vi "AO_arbitrary.vi"() -> ()   [LabVIEW 2021]
uses:
  <vilib>/userdefined/High Color/nirio_resource_hc.ctl
  <vilib>/FPGAPlugInAG/PCIe-7857/niLvFpga_Open_PCIe-7857.vi
  <vilib>/Utility/error.llb/Error Cluster From Error Code.vi
  <vilib>/rvi/errors/niLvFpgaAdjustHostInterfaceError.vi
  <vilib>/rvi/interface/common/niFpgaWaitOnOcc.vi
  <vilib>/FPGAPlugInAG/PCIe-7857/niLvFpga_Run_PCIe-7857.vi
  <vilib>/FPGAPlugInAG/PCIe-7857/niLvFpga_Close_PCIe-7857.vi
  <vilib>/rvi/interface/nirviOpenFPGA/nirviOpenFPGA.xnode
  FPGA Bitfiles/lvfpga2_FPGATarget_FPGA_J9MBVCOB9rw.lvbitx
  FPGA.vi
  <vilib>/rvi/interface/nirviReadWriteControl/nirviReadWriteControl.xnode
  <vilib>/rvi/interface/nirviMethod/nirviMethod.xnode
  <vilib>/rvi/interface/nirviCloseFPGA/nirviCloseFPGA.xnode
  <vilib>/rvi/errors/niLvFpgaMergeErrorWithErrorCode.vi
  <vilib>/measure/NI_MABase.lvlib
  <vilib>/FPGAPlugInAG/PCIe-7857/niLvFpga_WriteFifo_PCIe-7857.vi
  <vilib>/FPGAPlugInAG/PCIe-7857/niLvFpga_ConfigureFifo_PCIe-7857.vi
  NiFpgaLv.dll
panel:
  out "Actual Depth":u32
  out "Waveform Graph 2":dbl[](graph)
  out "Waveform Graph":waveform(dbl)(graph)
  in  "RIO Resource Name":T1="RIO0" caption="RIO Device"
  in  "Sample Clock Rate":dbl=20000.0 format="%0.2f"
  in  "stop":bool
  out "Actual Sample Clock Rate":dbl=20000.0 format="%.2f"
  in  "Size (Samples)":u32=5000
  in  "Waveform Type":T2(ring)
  in  "Frequency":sgl=997.0 format="%.2f"
  in  "Amplitude":sgl=1.0 format="%0.2p"
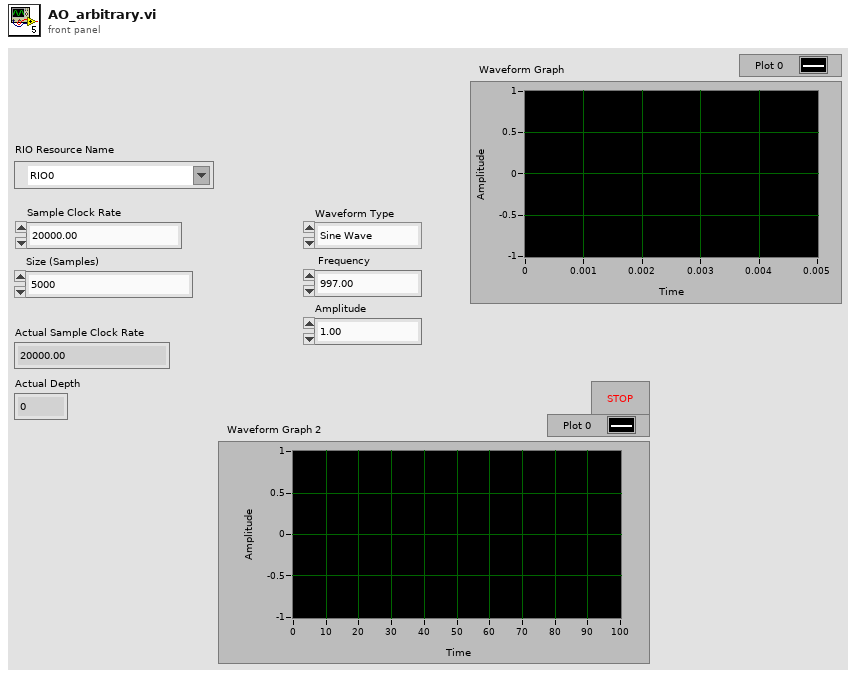
[diagram p1: front panel]
types:
  T1 = typedef "nirio_resource_hc.ctl" = tag
  T2 = enum16{"Sine Wave", "Triangle Wave", "Square Wave", "Sawtooth Wave"}
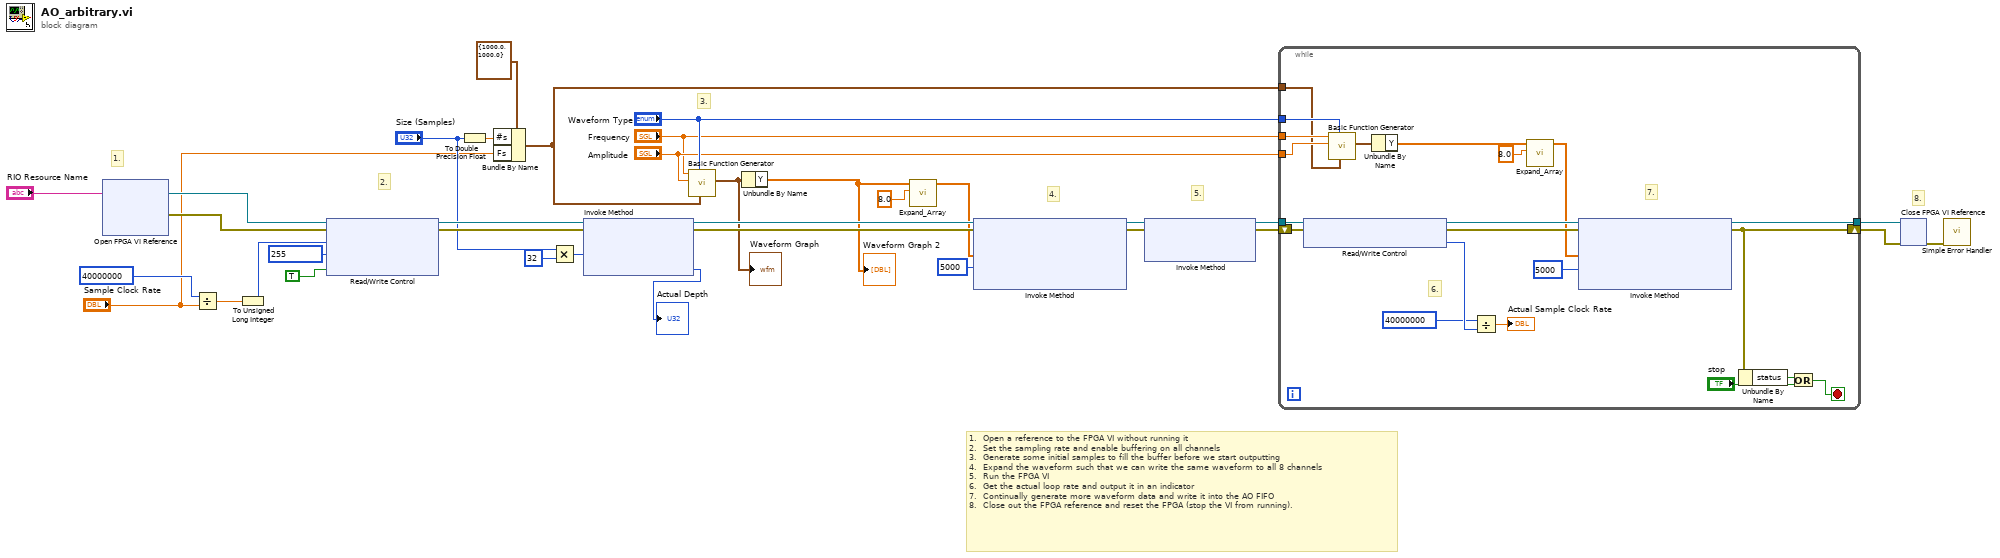
[diagram p0: block diagram]
diagram:
  # "1."
  # "1.  Open a reference to the FPGA VI without running it\n2.  Set the sampling rate and enable buffering on all channels\n3.  Generate some initial samples to fill the buffer before we start outputting\n4.  Expand the waveform such that we can write the same waveform to all 8 channels\n5.  Run the FPGA VI\n6.  Get the actual loop rate and output it in an indicator\n7.  Continually generate more waveform data and write it into the AO FIFO\n8.  Close out the FPGA reference and reset the FPGA (stop the VI from running)."
  # "8."
  # "5."
  # "4."
  # "3."
  # "2."
  n1 = xnode "Open FPGA VI Reference"("resource name"="RIO Resource Name") -> ("FPGA VI Reference Out"=w9:refnum<k20>, "error out"=w10:errorcluster)  [unwired: 1 in]
  n2 = Divide(x=u32 40000000, y="Sample Clock Rate") -> (x/y=w11:dbl)
  n3 = To Unsigned Long Integer(number=w11) -> (unsigned 32bit integer=w7:u32)
  n4 = xnode "Read/Write Control"("FPGA VI Reference In"=w9, "error in"=w10, "AO Loop Timer(us)"=w7, "AO Buffer Enable"=u8 255, "AO Enable"=TRUE) -> ("FPGA VI Reference Out"=w20:refnum<k20>, "error out"=w19:errorcluster)
  n5 = To Double Precision Float(number="Size (Samples)") -> (double precision float=w32:dbl)
  n6 = Bundle By Name(cluster=cluster{"Fs":dbl, "#s":dbl} {"Fs"=1000.0, "#s"=1000.0} ("sampling info"), "#s"=w32, "Fs"="Sample Clock Rate") -> (w27:cluster{"Fs":dbl, "#s":dbl})
  n7 = Multiply(x="Size (Samples)", y=u32 32) -> (x*y=w14:u32)
  n8 = xnode "Invoke Method"("FPGA VI Reference In"=w20, "error in"=w19, "Requested Depth"=w14) -> ("FPGA VI Reference Out"=w18:refnum<k20>, "error out"=w17:errorcluster, "Actual Depth"=→"Actual Depth":u32)
  n9 = call <vilib>:"Basic Function Generator.vi"("sampling info"=w27, "signal type"="Waveform Type", "amplitude"="Amplitude", "frequency"="Frequency") -> ("signal out"=w5:waveform(dbl))  [unwired: 5 in, 2 out]
  "Waveform Graph" <- w5
  n10 = Unbundle By Name(w5) -> ("Y"=w1:dbl[])
  "Waveform Graph 2" <- w1
  n11 = call "Expand_Array.vi"("Scale Factor"=sgl 8.0, "Input AO Array"=w1) -> ("Output Array"=w4:sgl[])  [unwired: 9 in]
  n12 = xnode "Invoke Method"("FPGA VI Reference In"=w18, "error in"=w17, "Data"=w4, "Timeout (ms)"=5000) -> ("FPGA VI Reference Out"=w30:refnum<k20>, "error out"=w21:errorcluster)  [unwired: 1 out]
  n13 = xnode "Invoke Method"("FPGA VI Reference In"=w30, "error in"=w21) -> ("FPGA VI Reference Out"=w29:refnum<k20>, "error out"=w28:errorcluster)  [unwired: 1 in]
  n14 = while {
    tunnel: w29 -> [w49]
    shift-right: [w40] -> w23
    shift-left: w28 -> [w48]
    tunnel: w27 -> [w53]
    tunnel: "Waveform Type" -> [w56]
    tunnel: "Frequency" -> [w55]
    tunnel: "Amplitude" -> [w54]
    tunnel: [w51] -> w24
    stop <- w41 stop-if-true
    # "7."
    # "6."
    n15 = xnode "Read/Write Control"("FPGA VI Reference In"=w49, "error in"=w48) -> ("FPGA VI Reference Out"=w47:refnum<k20>, "error out"=w46:errorcluster, "AO: Actual Loop Rate(us)"=w45:u32)
    n16 = call <vilib>:"Basic Function Generator.vi"("sampling info"=w53, "signal type"=w56, "amplitude"=w54, "frequency"=w55) -> ("signal out"=w52:waveform(dbl))  [unwired: 5 in, 2 out]
    n17 = Unbundle By Name(w52) -> ("Y"=w36:dbl[])
    n18 = Divide(x=u32 40000000, y=w45) -> (x/y=→"Actual Sample Clock Rate":dbl)
    n19 = call "Expand_Array.vi"("Scale Factor"=sgl 8.0, "Input AO Array"=w36) -> ("Output Array"=w37:sgl[])  [unwired: 9 in]
    n20 = xnode "Invoke Method"("FPGA VI Reference In"=w47, "error in"=w46, "Data"=w37, "Timeout (ms)"=5000) -> ("FPGA VI Reference Out"=w51:refnum<k20>, "error out"=w40:errorcluster)  [unwired: 1 out]
    n21 = Unbundle By Name(w40) -> ("status"=w39:bool)
    n22 = Or(x=w39, y="stop") -> (x .or. y?=w41:bool)
  }
  n23 = xnode "Close FPGA VI Reference"("FPGA VI Reference In"=w24, "error in"=w23) -> ("error out"=w22:errorcluster)
  n24 = call <vilib>:"Simple Error Handler.vi"("error in (no error)"=w22) -> ()  [unwired: 4 in, 5 out]
